vi "Day 18-Part 1.vi"() -> ()   [LabVIEW 2021]
uses:
  <vilib>/Utility/file.llb/Read Delimited Spreadsheet (string).vi
panel:
  out "Magnitude":i32
  out "Resulting Number":i32[][](array[numeric])
  out "Input":string[](array[string])
  in  "Input File":enum32{"example input", "input"}(radio)
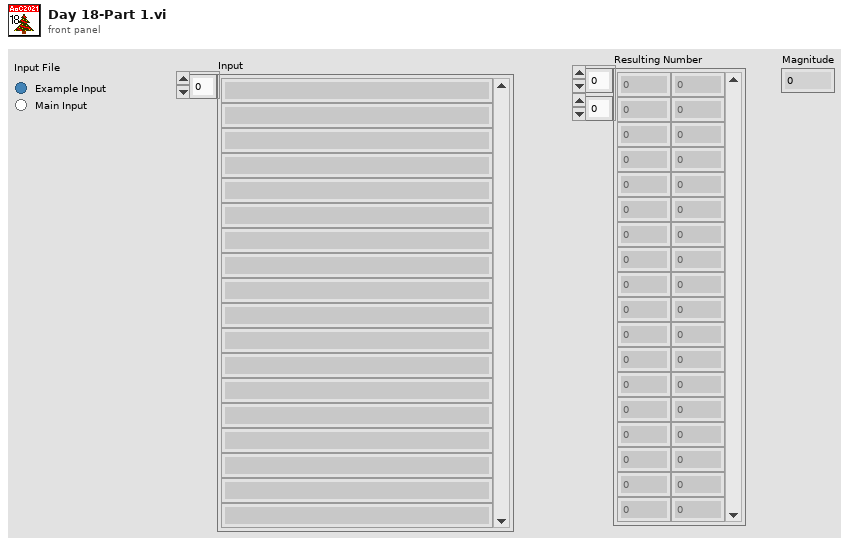
[diagram p1: front panel]
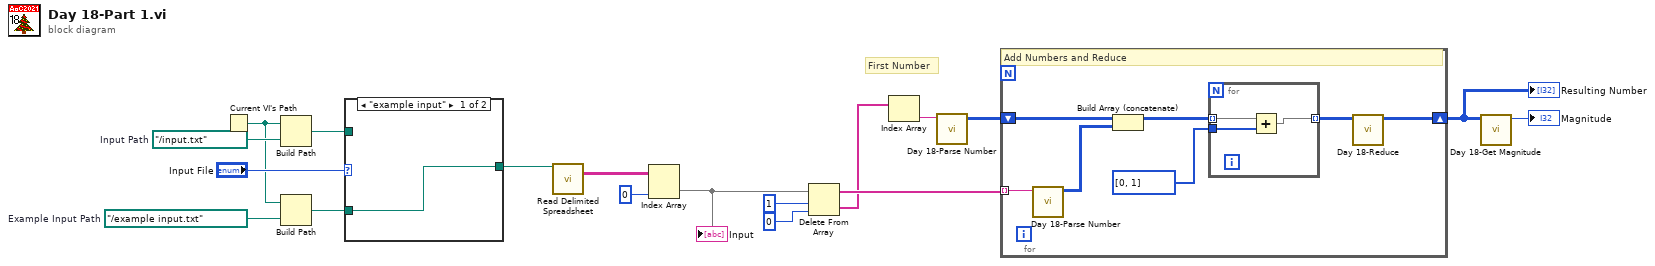
[diagram p0: block diagram]
diagram:
  w17 = path "../example input.txt"  # Example Input Path
  w18 = path "../input.txt"  # Input Path
  # "First Number"
  n1 = Current VI's Path() -> (path=w12:path)
  n2 = Build Path(base path=w12, name or relative path=w18) -> (appended path=w15:path)
  n3 = Build Path(base path=w12, name or relative path=w17) -> (appended path=w14:path)
  n4 = case shown="\"example input\"" "Input File" {
    tunnel: w15 -> [_ w20]
    tunnel: w14 -> [w19 _]
    tunnel: [w19 w20] -> w13
    frame "example input" {
    }
    frame "input" {
    }
  }
  n5 = call-poly <vilib>:"Read Delimited Spreadsheet.vi"("file path (dialog if empty)"=w13) -> ("all rows"=w11:string[][])  [unwired: 9 in, 5 out]
  n6 = Index Array(array=w11, index (col)=0 ("disabled index (col)")) -> (element=w3:string[])  [unwired: 1 in]
  "Input" <- w3
  n7 = Delete From Array(array=w3, length=1, index=0) -> (deleted portion=w6:string[], array with subset deleted=w7:string[])
  n8 = Index Array(array=w6) -> (element=w5:string)  [unwired: 1 in]
  n9 = call "Day 18-Parse Number.vi"("Data in"=w5) -> ("Data out"=w4:i32[][])  [unwired: 10 in]
  n10 = for {
    tunnel: w7 -> [w25] mode=indexing
    shift-right: [w26] -> w2
    shift-left: w4 -> [w24]
    # "Add Numbers and Reduce"
    n11 = call "Day 18-Parse Number.vi"("Data in"=w25) -> ("Data out"=w22:i32[][])  [unwired: 10 in]
    n12 = Build Array (concatenate)(w24, w22) -> (w23:i32[][])
    n13 = for {
      tunnel: w23 -> [w30] mode=indexing
      tunnel: i32[] [0, 1] -> [w29]
      tunnel: [w28] -> w21 mode=indexing
      n14 = Add(x=w30, y=w29) -> (x+y=w28:i32[])
    }
    n15 = call "Day 18-Reduce.vi"("Array in"=w21) -> ("Array out"=w26:i32[][])  [unwired: 10 in]
  }
  "Resulting Number" <- w2
  n16 = call "Day 18-Get Magnitude.vi"("Array in"=w2) -> ("Magnitude"=→"Magnitude":i32)  [unwired: 10 in]
